vi "set_data_for_channel.vi"(8 "error in (no error)":errorcluster, 10 "data":dbl[](array[numeric]), 11 "GenericWriteSignals in":refnum<class "GenericSignalWriter.lvclass">) -> (0 "error out":errorcluster, 3 "GenericWriteSignals out":refnum<class "GenericSignalWriter.lvclass">)   [LabVIEW 2010, in "GenericSignalWriter.lvclass"]
uses:
  GenericSignalWriter.lvclass
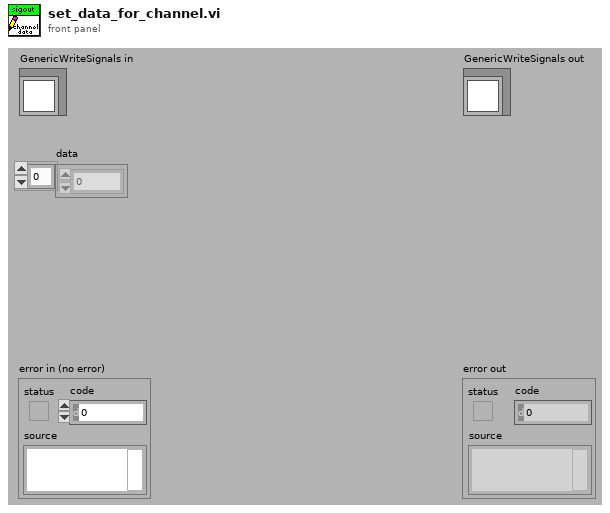
[diagram p1: front panel]
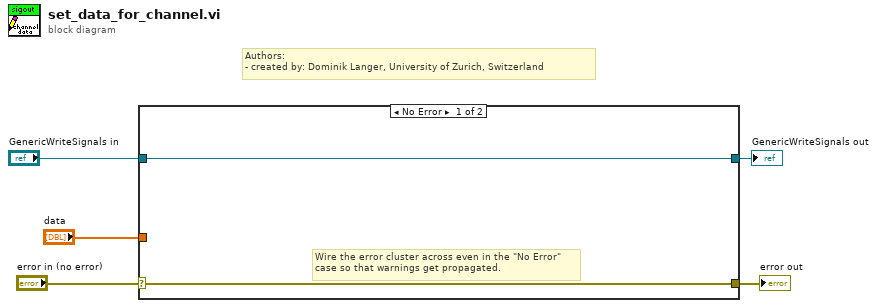
[diagram p0: block diagram]
diagram:
  # "Authors: \n- created by: Dominik Langer, University of Zurich, Switzerland"
  n1 = case shown="No Error" "error in (no error)" {
    selector: "error in (no error)" -> [w6 w9]
    tunnel: [w6 w9] -> w4
    tunnel: [w7 w8] -> w2
    tunnel: "GenericWriteSignals in" -> [w7 w8]
    tunnel: "data" -> [_ _]
    frame No Error {
      # "Wire the error cluster across even in the \"No Error\"\ncase so that warnings get propagated."
    }
    frame Error {
    }
  }
  "error out" <- w4
  "GenericWriteSignals out" <- w2
